vi "LoadLogCounter.vi"   [LabVIEW 2013]
uses:
  Global.vi
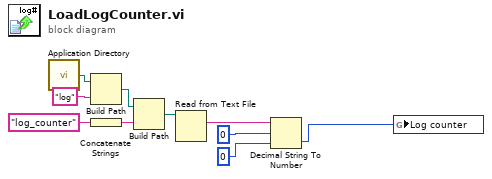
[diagram p0: block diagram]
diagram:
  n1 = call <vilib>:"Application Directory.vi"() -> ("Application Directory"=w8:path)
  n2 = Build Path(base path=w8, name or relative path="log") -> (appended path=w6:path)
  n3 = Concatenate Strings("log_counter" ("string")) -> (w4:string)
  n4 = Build Path(base path=w6, name or relative path=w4) -> (appended path=w9:path)
  n5 = Read from Text File(file (use dialog)=w9) -> (text=w10:string)  [unwired: 3 in, 3 out]
  n6 = Decimal String To Number(string=w10, offset=0, default (0L)=0 ("default (0 I32)")) -> (number=w1:i32)  [unwired: 1 out]
  n7 = global write "Global.vi" "Log counter"(w1) -> ()
